vi "PI Convert 1.6 to 1.7.vi"(0 "Prompted Inputs 1.6 Test Parameters":T2) -> (2 "Prompted Inputs 1.7 Test Parameters":T1)   [LabVIEW 2011]
uses:
  TypeDefs/PI Test Parameters v1.6.ctl
  TypeDefs/PI Test Parameters v1.7.ctl
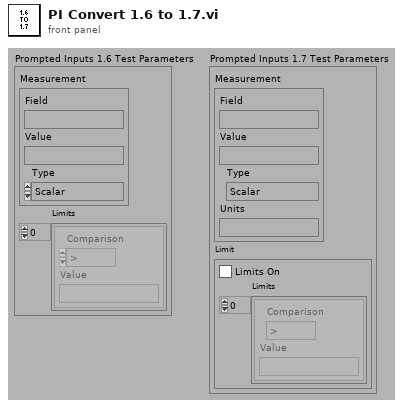
[diagram p1: front panel]
types:
  T1 = typedef "PI Test Parameters v1.7.ctl" = cluster{"Measurement":cluster{"Field":string, "Value":string, "Type":enum16{"Scalar", "Enumeration"}, "Units":string}, "Limit":cluster{"Limits On":bool, "Limits":cluster{"Comparison":enum16{">", ">=", "<", "<=", "<>", "="}, "Value":string}[]}}
  T2 = typedef "PI Test Parameters v1.6.ctl" = cluster{"Measurement":cluster{"Field":string, "Value":string, "Type":enum16{"Scalar", "Enumeration"}}, "Limits":cluster{"Comparison":enum16{">", ">=", "<", "<=", "<>", "="}, "Value":string}[]}
  T3 = cluster{"Comparison":enum16{">", ">=", "<", "<=", "<>", "="}, "Value":string}[]
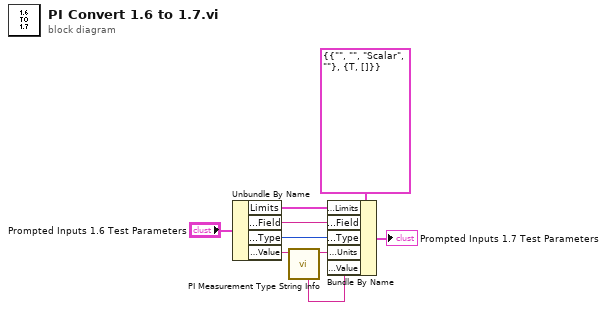
[diagram p0: block diagram]
diagram:
  n1 = Unbundle By Name("Prompted Inputs 1.6 Test Parameters") -> ("Limits"=w6:T3, "Measurement.Field"=w5:string, "Measurement.Type"=w4:enum16{"Scalar", "Enumeration"}, "Measurement.Value"=w3:string)
  n2 = call "PI Measurement Type String Info.vi"("Prompt Measurement Type String"=w3) -> ("comma list"=w1:string, "Units (Scalar)"=w2:string)  [unwired: 9 out]
  n3 = Bundle By Name(cluster=T1 {"Measurement"={"Field"="", "Value"="", "Type"=enum."Scalar", "Units"=""}, "Limit"={"Limits On"=TRUE, "Limits"=[]}} ("Prompted Inputs Test Parameters"), "Limit.Limits"=w6, "Measurement.Field"=w5, "Measurement.Type"=w4, "Measurement.Units"=w2, "Measurement.Value"=w1) -> (→"Prompted Inputs 1.7 Test Parameters":T1)
